vi "ITR LP.vi"(7 "input":dbl format="%.2f", 13 "corner period (steps)":dbl(slide)=10.237739663395852 scale=1.0..1000.0) -> (8 "output":dbl format="%.2f")   [LabVIEW 2016]
doc: "Modular ITR first order low pass filter with internal shift registers."
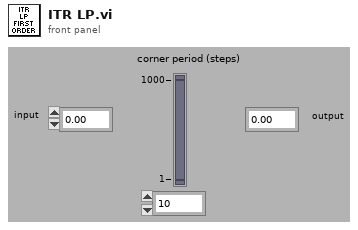
[diagram p1: front panel]
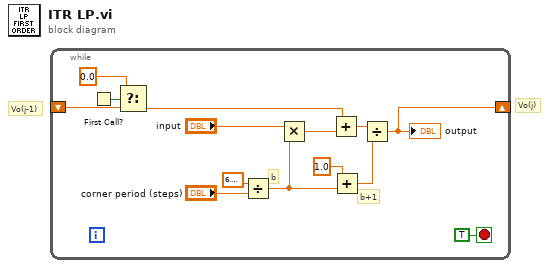
[diagram p0: block diagram]
diagram:
  # "Vo(j-1)"
  # "Vo(j)"
  n1 = while {
    shift-left: _ -> [w4]
    shift-right: [w6] -> _
    stop <- TRUE stop-if-true
    # "b+1"
    # "b"
    n2 = First Call?() -> (First Call?: T/F=w1:bool)
    n3 = Select(t=0.0, s=w1, f=w4) -> (s? t:f=w3:dbl)
    n4 = Divide(x=6.283185307179586, y="corner period (steps)") -> (x/y=w9:dbl)
    n5 = Multiply(x="input", y=w9) -> (x*y=w5:dbl)
    n6 = Add(x=w3, y=w5) -> (x+y=w8:dbl)
    n7 = Add(x=1.0, y=w9) -> (x+y=w7:dbl)
    n8 = Divide(x=w8, y=w7) -> (x/y=w6:dbl)
    "output" <- w6
  }
